vi "Fill Maps.vi"(11 "Project In":refnum<class "Project.lvclass">) -> (2 "Tree Map out":T1, 3 "Project Out":refnum<class "Project.lvclass">)   [LabVIEW 2019, in "Panther Dashboard.lvlib"]
uses:
  Panther Dashboard.lvlib
  <vilib>/National Instruments/Tree Map/Tree Map Data.ctl
  <vilib>/National Instruments/Tree Map/Tree Map.lvlib
  Map Attribute--enum.ctl
  Class/Project/Project.lvclass
  Class/Library/Library.lvclass
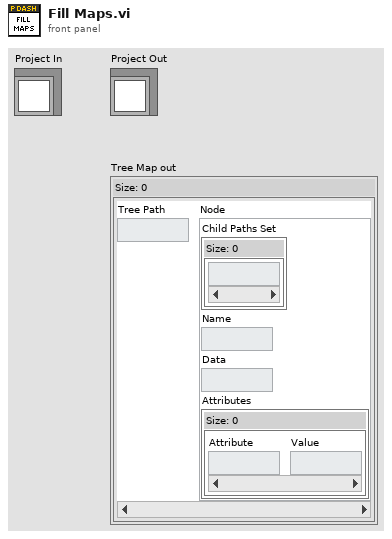
[diagram p1: front panel]
types:
  T1 = typedef "Tree Map.lvlib/Tree Map Data.ctl" = map{string, cluster{"Child Paths Set":set{string}, "Name":string, "Data":string, "Attributes":map{string, string}}}
  T2 = typedef "Panther Dashboard.lvlib/Map Attribute--enum.ctl" = enum16{"Path", "ModuleType", "Module Description", "Dependency?", "Target"}
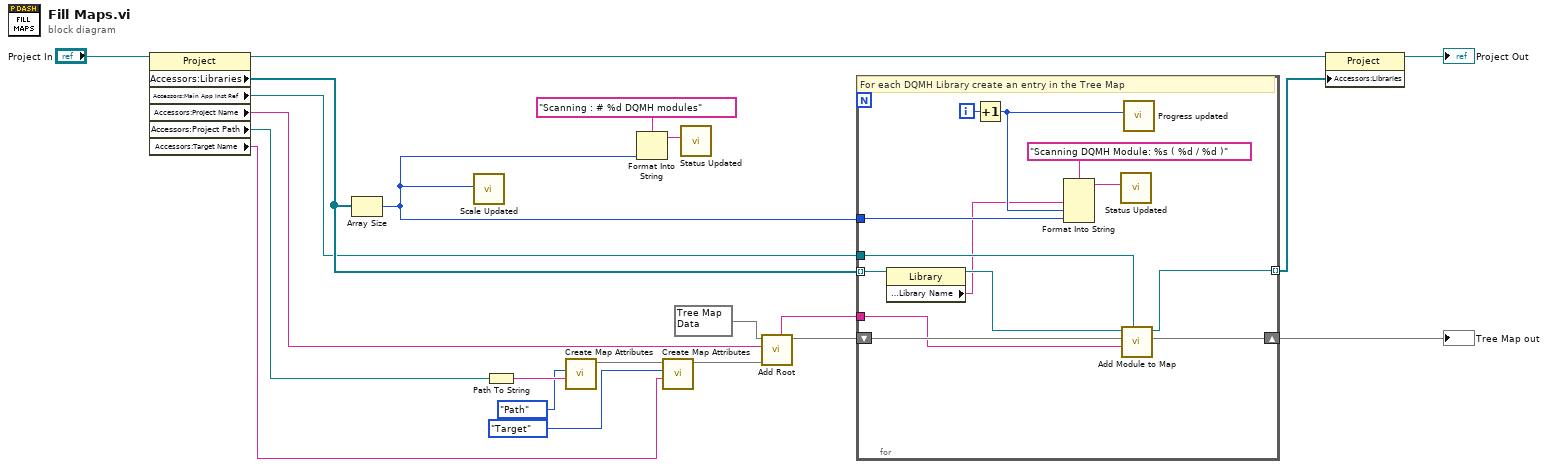
[diagram p0: block diagram]
diagram:
  n1 = property class="Project"(reference="Project In") -> (reference out=w7:refnum<class "Project.lvclass">, "Accessors:Libraries"=w8:refnum<class "Library.lvclass">[], "Accessors:Main App Inst Ref"=w4:refnum<vi>, "Accessors:Project Name"=w3:string, "Accessors:Project Path"=w2:path, "Accessors:Target Name"=w1:string)  [unwired: 1 in, 1 out]
  n2 = Array Size(array=w8) -> (size(s)=w18:i32)
  n3 = call "Scale Updated.vi"("Scale Max"=w18) -> ()  [unwired: 10 in, 1 out]
  n4 = Path To String(path=w2) -> (string=w14:string)
  n5 = call "Create Map Attributes.vi"("Attribute"=w14, "Map Attribute"=Map_Attribute--enum."Path") -> ("Root Attributes"=w12:map{string, string})  [unwired: 9 in]
  n6 = Format Into String(format string="Scanning : # %d DQMH modules", w18) -> (resulting string=w21:string)  [unwired: 2 in, 1 out]
  n7 = call "Create Map Attributes.vi"("Attribute"=w1, "Map Attribute"=Map_Attribute--enum."Target", "Root Attributes In"=w12) -> ("Root Attributes"=w11:map{string, string})  [unwired: 8 in]
  n8 = call "Status Updated.vi"("Status"=w21) -> ()  [unwired: 10 in, 1 out]
  n9 = call <vilib>:"Add Root.vi"("Root Attributes"=w11, "New Root Name"=w3, "Tree Map In"=T1 {} ("Tree Map out")) -> ("Tree Map Out"=w17:T1, "Root Path"=w16:string)  [unwired: 7 in]
  n10 = for {
    shift-right: [w34] -> w19
    shift-left: w17 -> [w28]
    tunnel: w18 -> [w32]
    tunnel: w4 -> [w27]
    tunnel: w16 -> [w24]
    tunnel: w8 -> [w26] mode=indexing
    tunnel: [w25] -> w5 mode=indexing
    i -> [w33]
    # "For each DQMH Library create an entry in the Tree Map"
    n11 = property class="Library"(reference=w26) -> (reference out=w23:refnum<class "Library.lvclass">, "Accessors:Library Name"=w22:string)  [unwired: 1 in, 1 out]
    n12 = Increment(x=w33) -> (x+1=w29:i32)
    n13 = Format Into String(format string="Scanning DQMH Module: %s ( %d / %d )", w22, w29, w32) -> (resulting string=w30:string)  [unwired: 2 in, 1 out]
    n14 = call "Status Updated.vi"("Status"=w30) -> ()  [unwired: 10 in, 1 out]
    n15 = call "Add Module to Map.vi"("App Ref"=w27, "Parent Path"=w24, "Tree Map in"=w28, "Library In"=w23) -> ("Tree Map out"=w34:T1, "Library Out"=w25:refnum<class "Library.lvclass">)  [unwired: 6 in]
    n16 = call "Progress updated.vi"("Progress"=w29) -> ()  [unwired: 10 in, 1 out]
  }
  "Tree Map out" <- w19
  n17 = property class="Project"(reference=w7, "Accessors:Libraries"=w5) -> (reference out=→"Project Out":refnum<class "Project.lvclass">)  [unwired: 1 in, 1 out]
